vi "TSM Apply Digital Levels Timing.vi"(0 "TSM context":T1, 5 "Levels Sheet":string, 7 "Timing Sheet":string, 11 "error in":errorcluster) -> (15 "error out":errorcluster)   [LabVIEW 2020]
uses:
  <vilib>/NI_TestStand_SemiconductorModule/NI_TestStand_Semiconductor_Module.lvlibp/PinMap/General/SemiconductorModuleContext.ctl
  <vilib>/NI_TestStand_SemiconductorModule/NI_TestStand_Semiconductor_Module.lvlibp
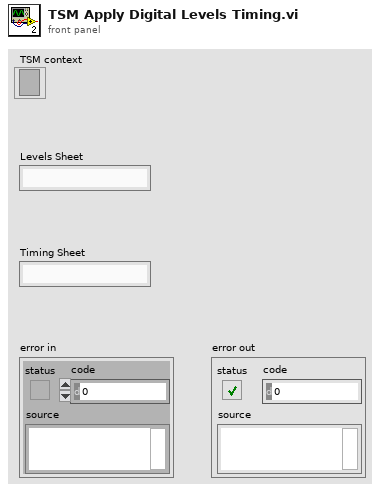
[diagram p1: front panel]
types:
  T1 = typedef "NI_TestStand_Semiconductor_Module.lvlibp/SemiconductorModuleContext.ctl" = refnum<k7>
  T2 = typedef "TSM SSC Digital.ctl" = cluster{"Pin Query Context":refnum<class "DigitalPatternPinQueryContext.lvclass">, "SSC":T3[], "Site Numbers":i32[], "Pins":tag[]}
  T3 = typedef "SSC Digital.ctl" = cluster{"Session":refnum<k15>, "Channel List":string, "Site List":string}
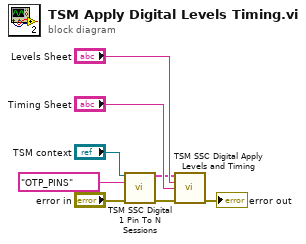
[diagram p0: block diagram]
diagram:
  n1 = call "TSM SSC Digital 1 Pin To N Sessions.vi"("TSM context"="TSM context", "Pin"=tag "OTP_PINS", "error in"="error in") -> ("Digital TSM Out"=w6:T2, "error out"=w5:errorcluster)  [unwired: 11 in]
  n2 = call "TSM SSC Digital Apply Levels and Timing.vi"("Digital TSM In"=w6, "Levels Sheet"="Levels Sheet", "Timing Sheet"="Timing Sheet", "error in"=w5) -> ("error out"=→"error out":errorcluster)  [unwired: 10 in, 1 out]
